vi "Tutorial 10.vi"() -> ()   [LabVIEW 2014]
panel:
  out "Sum":dbl
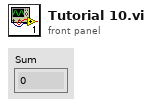
[diagram p1: front panel]
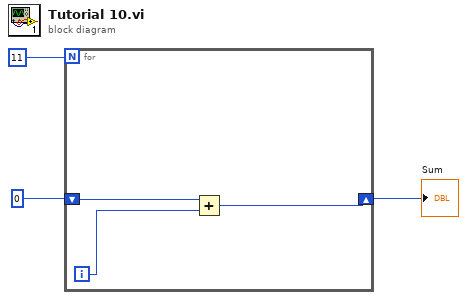
[diagram p0: block diagram]
diagram:
  n1 = for {
    N: 11 -> [_]
    shift-right: [w5] -> w1
    shift-left: 0 -> [w4]
    i -> [w6]
    n2 = Add(x=w4, y=w6) -> (x+y=w5:i32)
  }
  "Sum" <- w1
